vi "Gs to fps^2.vi"(10 "g":dbl) -> (2 "f/s^2":dbl)   [LabVIEW 2015]
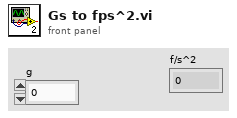
[diagram p1: front panel]
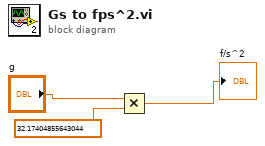
[diagram p0: block diagram]
diagram:
  n1 = Multiply(x="g", y=32.17404855643044) -> (x*y=→"f/s^2":dbl)
